vi "FGV Simple Register and Unregister.vi"() -> (2 "response message":string[](array[string]), 3 "response message":string[](array[string]))   [LabVIEW 2017, in "testcase-Broadcast Registry.lvclass"]
uses:
  testcase-Broadcast Registry.lvclass
  src/user.lib/_NEVSTOP/Communicable State Machine(CSM)/_Support/FGV-BroadcastRegistry/Operation-BroadcastRegistry.ctl
  src/user.lib/_NEVSTOP/Communicable State Machine(CSM)/Communicable State Machine.lvlib
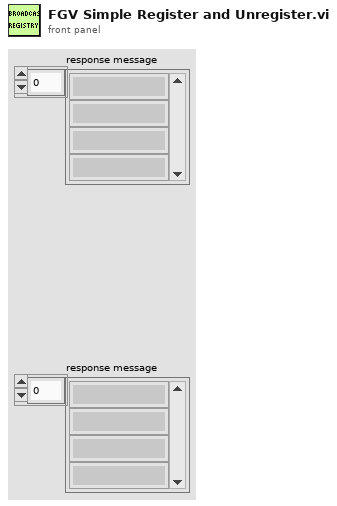
[diagram p1: front panel]
types:
  T1 = typedef "Communicable State Machine.lvlib/Operation-BroadcastRegistry.ctl" = enum16{"Delete Source Module", "Delete Target Module", "Remove Module", "Register", "Unregister", "Check", "List Status", "List Entries", "List Status Of Source", "Drop", "Register As Status", "Register As Interrupt"}
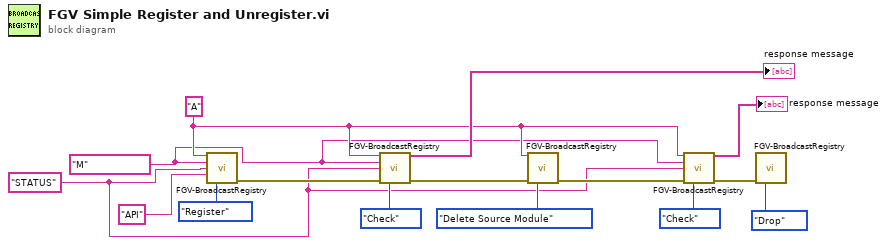
[diagram p0: block diagram]
diagram:
  w4 = "STATUS" ("Message")
  w5 = "M" ("Dest")
  w6 = "A" ("Source")
  n1 = call "FGV-BroadcastRegistry.vi"("Source"=w6, "Target"=w5, "Status"=w4, "API"="API" ("Response Message In"), "Operation"=Operation-BroadcastRegistry."Register") -> ("error out"=w13:errorcluster)  [unwired: 8 in, 2 out]
  n2 = call "FGV-BroadcastRegistry.vi"("Source"=w6, "Target"=w5, "Status"=w4, "Error In"=w13, "Operation"=Operation-BroadcastRegistry."Check") -> ("Response Message"=→"response message":string[], "error out"=w10:errorcluster)  [unwired: 8 in, 1 out]
  n3 = call "FGV-BroadcastRegistry.vi"("Source"=w6, "Error In"=w10, "Operation"=Operation-BroadcastRegistry."Delete Source Module") -> ("error out"=w7:errorcluster)  [unwired: 10 in, 2 out]
  n4 = call "FGV-BroadcastRegistry.vi"("Source"=w6, "Target"=w5, "Status"=w4, "Error In"=w7, "Operation"=Operation-BroadcastRegistry."Check") -> ("Response Message"=→"response message":string[], "error out"=w2:errorcluster)  [unwired: 8 in, 1 out]
  n5 = call "FGV-BroadcastRegistry.vi"("Error In"=w2, "Operation"=Operation-BroadcastRegistry."Drop") -> ()  [unwired: 11 in, 3 out]
